vi "SPI Master and Slave with debug using PXI Trig [FPGA].vi"() -> ()   [LabVIEW 2019]
uses:
  <vilib>/Platform/TimedLoop/XDataNode/timing_clust.ctl
  <vilib>/Platform/TimedLoop/XDataNode/nitl_modes.ctl
  <vilib>/Platform/TimedLoop/XDataNode/wakeup.ctl
  SPI Master State.ctl
  SPI Slave State.ctl
  <vilib>/rvi/Emulation/niFpgaSctlEmulationGetInTimedLoop.vi
  <vilib>/rvi/Emulation/niFpgaEmulationReportErrorSimple.vi
  <vilib>/rvi/Emulation/niFpgaGetClockAttributes.vi
  <vilib>/rvi/Emulation/niFpgaCriticalErrorInLSC.vi
  <vilib>/rvi/eio/common/nirviEmuTemplateMethod_errors.vi
  <vilib>/rvi/interface/RandomDataEmulation/niFpgaRandomDataHandleErrors.vi
  <vilib>/Platform/TimedLoop/XDataNode/XDataNode.xnode
  <vilib>/eio/EIONode/EIONode.xnode
  <vilib>/rvi/DataTransferAndStorage/Container/XNode/niFpgaContainer.xnode
  <vilib>/rvi/interface/RandomDataEmulation/nirviRandomDataFpgaReadWriteTemplate.vi
  <vilib>/Platform/TimedLoop/XDataNode/XDNodeRunTimeDep.lvlib
panel:
  out "Slave Data Out":u32
  in  "Slave Data In":u32
  in  "Data Length":u8
  in  "HCP-1":u8
  out "Data Out":u32
  in  "Data In":u32
  in  "TX":bool
  in  "CPOL":bool
  in  "CPHA":bool
  in  "RESET":bool
  out "MISO":bool
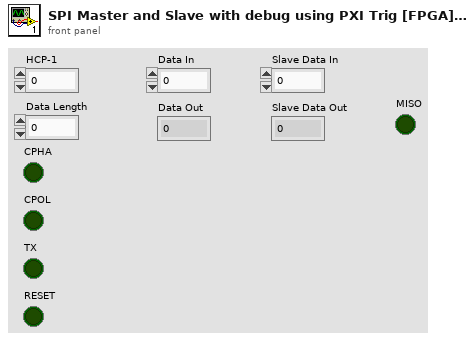
[diagram p1: front panel]
types:
  T1 = typedef "XDNodeRunTimeDep.lvlib/timing_clust.ctl" = cluster{"Expected End [f-1]":u64, "Actual End [f-1]":u64, "Finished Late? [f-1]":bool, "Expected End [i-1]":u64, "Actual End [i-1]":u64, "Finished Late? [i-1]":bool, "Expected Start [i]":u64, "Actual Start [i]":u64, "Expected Start [f]":u64, "Actual Start [f]":u64, "Source Name":string, "Structure Name":string, "Period":i64, "Deadline":i64, "Offset":i64, "Start":i64, "Priority":i32, "Timeout":i32, "Mode":T2, "Wakeup Reason":T3, "Error":errorcluster, "Source Type":string, "Secondary Source Type":string, "Global End Time":u64, "Global Start Time":u64, "Frame Duration":u64, "Iteration Duration":u64, "Assigned CPU":i32, "I/O Scan Engine Mode":u32}
  T2 = typedef "XDNodeRunTimeDep.lvlib/nitl_modes.ctl" = enum32{"No Change", "Process missed periods, maintain original phase", "Discard missed periods, maintain original phase", "Process missed periods, ignore original phase", "Discard missed periods, ignore original phase"}
  T3 = typedef "XDNodeRunTimeDep.lvlib/wakeup.ctl" = enum32{"Normal", "Aborted", "Asynchronous wakeup", "Timing source error", "Timed loop error", "Timeout"}
  T4 = typedef "SPI Slave State.ctl" = enum8{"RESET", "Wait for _SS", "Assert MISO", "Latch MOSI"}
  T5 = typedef "SPI Master State.ctl" = enum8{"RESET", "Wait for TX", "Assert MOSI", "Toggle SCLK", "Latch MISO and Toggle SCLK", "Assert MOSI and Toggle SCLK"}
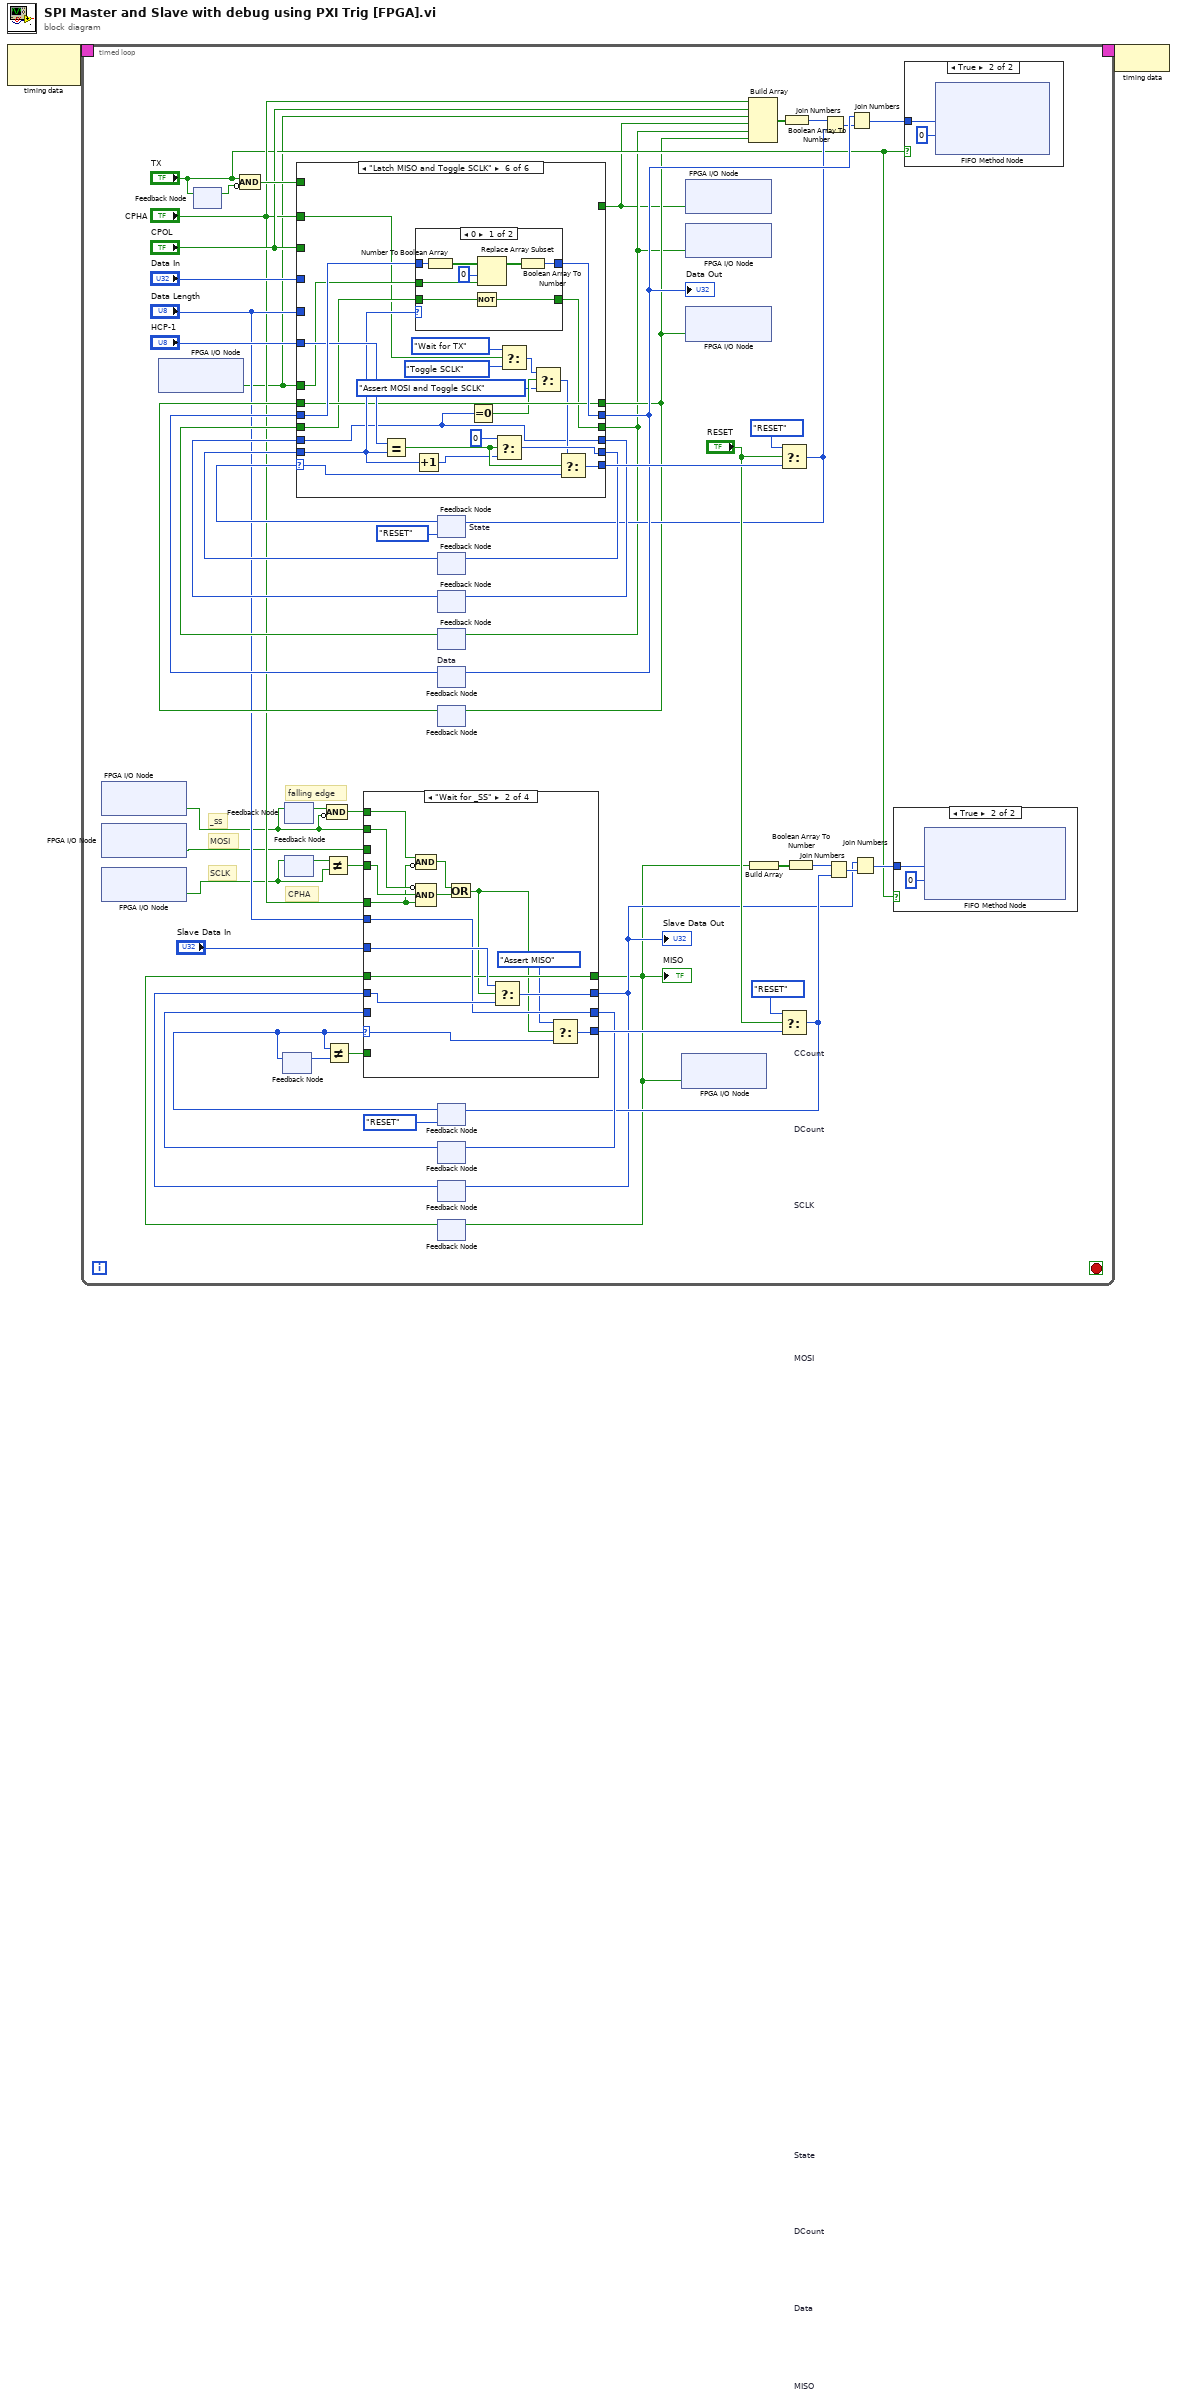
[diagram p0: block diagram]
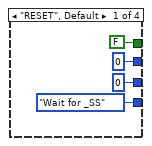
[diagram p3: hidden frame]
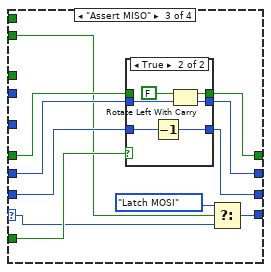
[diagram p4: hidden frame]
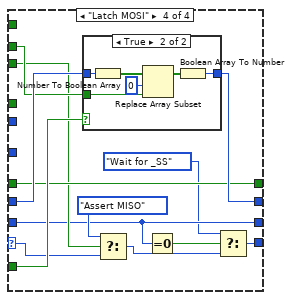
[diagram p6: hidden frame]
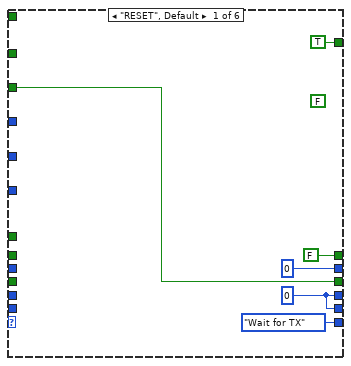
[diagram p9: hidden frame]
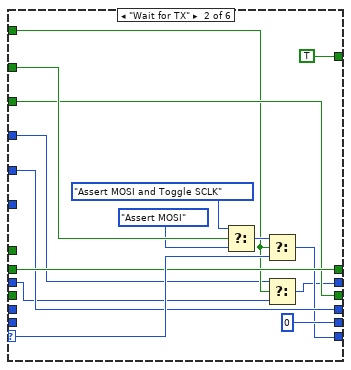
[diagram p10: hidden frame]
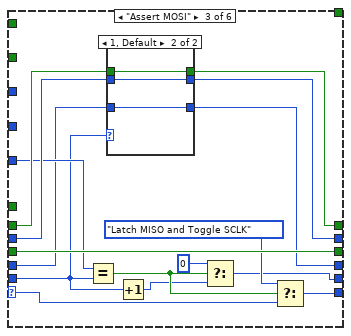
[diagram p11: hidden frame]
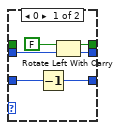
[diagram p12: hidden frame]
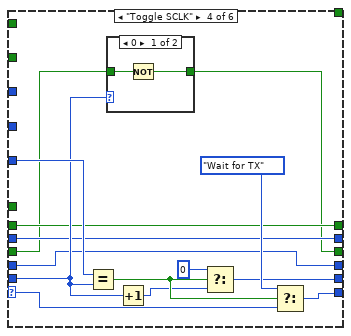
[diagram p13: hidden frame]
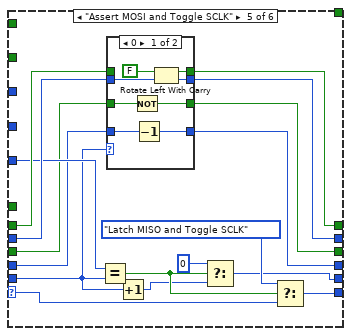
[diagram p15: hidden frame]
diagram:
  n1 = node-c288() -> (w2:T1)  [unwired: 1 in]
  n2 = timed-loop {
    timing: w2 -> [_]
    timing-out: [_] -> w1
    stop <- _ stop-if-true
    # "CPHA"
    # "falling edge"
    # "SCLK"
    # "MOSI"
    # "_SS"
    n3 = xnode "FPGA I/O Node"() -> ("PXI_Trig0"=w5:bool)  [unwired: 1 in, 1 out]
    n4 = xnode "FPGA I/O Node"() -> ("PXI_Trig2"=w4:bool)  [unwired: 1 in, 1 out]
    n5 = xnode "FPGA I/O Node"() -> ("PXI_Trig1"=w3:bool)  [unwired: 1 in, 1 out]
    n6 = xnode "FPGA I/O Node"() -> ("PXI_Trig3"=w9:bool)  [unwired: 1 in, 1 out]
    n7 = feedback #1() -> (w53:bool)  [unwired: 1 in]
    n8 = feedback-in #1("TX") -> ()
    n9 = Compound Arithmetic op=AND("TX", invert w53) -> (w45:bool)
    n10 = feedback #2 ("State")() -> (w20:T4)  [unwired: 1 in]
    n11 = feedback #3() -> (w24:bool)  [unwired: 1 in]
    n12 = feedback-in #3(w5) -> ()
    n13 = feedback #4() -> (w22:bool)  [unwired: 1 in]
    n14 = feedback-in #4(w3) -> ()
    n15 = Not Equal?(x=w22, y=w3) -> (x != y?=w21:bool)
    n16 = Compound Arithmetic op=AND(w24, invert w5) -> (w23:bool)
    n17 = feedback #5 "State"(SPI_Master_State."RESET") -> (w56:T5)
    n18 = feedback #6 "CCount"() -> (w50:u8)  [unwired: 1 in]
    n19 = feedback #7 "DCount"() -> (w49:u8)  [unwired: 1 in]
    n20 = feedback #8 "SCLK"() -> (w48:bool)  [unwired: 1 in]
    n21 = feedback #9 "Data"() -> (w46:u32)  [unwired: 1 in]
    n22 = feedback #10 "MOSI"() -> (w44:bool)  [unwired: 1 in]
    n23 = case shown="\"Latch MISO and Toggle SCLK\"" w56 {
      selector: w56 -> [_ w138 w150 w178 w194 w230]
      tunnel: [SPI_Master_State."Wait for TX" w131 w151 w179 w195 w231] -> w55
      tunnel: w45 -> [_ w130 _ _ _ _]
      tunnel: [w125 u8 0 w144 w172 w188 w225] -> w52
      tunnel: [w125 w133 w142 w171 w184 w213] -> w51
      tunnel: w50 -> [_ _ w147 w175 w191 w228]
      tunnel: w49 -> [_ _ w143 w171 w185 w213]
      tunnel: [TRUE ("MOSI") TRUE ("MOSI") _ _ _ _] -> w6
      tunnel: "CPHA" -> [_ w139 _ _ _ w219]
      tunnel: [w123 w132 w153 w167 w186 w221] -> w7
      tunnel: "CPOL" -> [w123 w132 _ _ _ _]
      tunnel: w48 -> [_ _ w153 w168 w187 w222]
      tunnel: "Data In" -> [_ w129 _ _ _ _]
      tunnel: [u32 0 ("Data In") w127 w156 w170 w199 w233] -> w38
      tunnel: w46 -> [_ w128 w157 w170 w200 w234]
      tunnel: "HCP-1" -> [_ _ w152 w180 w196 w232]
      tunnel: w9 -> [_ _ _ _ _ w223]
      tunnel: "Data Length" -> [_ w133 _ _ _ _]
      tunnel: [FALSE ("msb carry out") w134 w155 w169 w198 w224] -> w8
      tunnel: w44 -> [_ w134 w154 w169 w197 w224]
      frame "RESET", Default {
        (unwired) FALSE ("msb carry out")
        w125 = u8 0
      }
      frame "Wait for TX" {
        n24 = Select(t=SPI_Master_State."Assert MOSI and Toggle SCLK", s=w139, f=SPI_Master_State."Assert MOSI" ("t")) -> (s? t:f=w135:T5)
        n25 = Select(t=w135, s=w130, f=w138) -> (s? t:f=w131:T5)
        n26 = Select(t=w129, s=w130, f=w128) -> (s? t:f=w127:u32)
      }
      frame "Assert MOSI" {
        n27 = Equal?(x=w152, y=w147) -> (x = y?=w148:bool)
        n28 = case shown="1, Default" w147 {
          tunnel: w157 -> [w162 w165]
          tunnel: [w161 w165] -> w156
          tunnel: [w160 w166] -> w155
          tunnel: w154 -> [_ w166]
          tunnel: w143 -> [w159 w164]
          tunnel: [w158 w164] -> w142
          frame 0 {
            n29 = Decrement(x=w159) -> (x-1=w158:u8)
            n30 = Rotate Left With Carry(2:w162, 3:FALSE ("carry")) -> (0:w161:u32, 1:w160:bool)
          }
          frame 1, Default {
          }
        }
        n31 = Increment(x=w147) -> (x+1=w146:u8)
        n32 = Select(t=u8 0, s=w148, f=w146) -> (s? t:f=w144:u8)
        n33 = Select(t=SPI_Master_State."Latch MISO and Toggle SCLK", s=w148, f=w150) -> (s? t:f=w151:T5)
      }
      frame "Toggle SCLK" {
        n34 = Equal?(x=w180, y=w175) -> (x = y?=w176:bool)
        n35 = case shown="0" w175 {
          tunnel: w168 -> [w182 w183]
          tunnel: [w181 w183] -> w167
          frame 0 {
            n36 = Not(x=w182) -> (.not. x?=w181:bool)
          }
          frame 1, Default {
          }
        }
        n37 = Increment(x=w175) -> (x+1=w174:u8)
        n38 = Select(t=u8 0, s=w176, f=w174) -> (s? t:f=w172:u8)
        n39 = Select(t=SPI_Master_State."Wait for TX", s=w176, f=w178) -> (s? t:f=w179:T5)
      }
      frame "Assert MOSI and Toggle SCLK" {
        n40 = Equal?(x=w196, y=w191) -> (x = y?=w192:bool)
        n41 = case shown="0" w191 {
          tunnel: w200 -> [w207 w211]
          tunnel: [w206 w211] -> w199
          tunnel: [w205 w212] -> w198
          tunnel: w197 -> [_ w212]
          tunnel: w187 -> [w204 w210]
          tunnel: [w203 w210] -> w186
          tunnel: w185 -> [w202 w209]
          tunnel: [w201 w209] -> w184
          frame 0 {
            n42 = Not(x=w204) -> (.not. x?=w203:bool)
            n43 = Decrement(x=w202) -> (x-1=w201:u8)
            n44 = Rotate Left With Carry(2:w207, 3:FALSE ("carry")) -> (0:w206:u32, 1:w205:bool)
          }
          frame 1, Default {
          }
        }
        n45 = Increment(x=w191) -> (x+1=w190:u8)
        n46 = Select(t=u8 0, s=w192, f=w190) -> (s? t:f=w188:u8)
        n47 = Select(t=SPI_Master_State."Latch MISO and Toggle SCLK", s=w192, f=w194) -> (s? t:f=w195:T5)
      }
      frame "Latch MISO and Toggle SCLK" {
        n48 = Equal?(x=w232, y=w228) -> (x = y?=w229:bool)
        n49 = Increment(x=w228) -> (x+1=w227:u8)
        n50 = case shown="0" w228 {
          tunnel: w234 -> [w242 w244]
          tunnel: [w237 w244] -> w233
          tunnel: w223 -> [w240 _]
          tunnel: w222 -> [w236 w243]
          tunnel: [w235 w243] -> w221
          frame 0 {
            n51 = Number To Boolean Array(number=w242) -> (Boolean array=w241:bool[])
            n52 = Not(x=w236) -> (.not. x?=w235:bool)
            n53 = Replace Array Subset(array=w241, new element=w240, index=0) -> (w238:bool[])
            n54 = Boolean Array To Number(Boolean array=w238) -> (number=w237:u32)
          }
          frame 1, Default {
          }
        }
        n55 = Equal To 0?(x=w213) -> (x = 0?=w220:bool)
        n56 = Select(t=u8 0, s=w229, f=w227) -> (s? t:f=w225:u8)
        n57 = Select(t=SPI_Master_State."Wait for TX", s=w219, f=SPI_Master_State."Toggle SCLK" ("t")) -> (s? t:f=w215:T5)
        n58 = Select(t=w215, s=w220, f=SPI_Master_State."Assert MOSI and Toggle SCLK" ("t")) -> (s? t:f=w217:T5)
        n59 = Select(t=w217, s=w229, f=w230) -> (s? t:f=w231:T5)
      }
    }
    "Data Out" <- w38
    n60 = feedback-in #6(w52) -> ()
    n61 = feedback-in #7(w51) -> ()
    n62 = feedback-in #8(w7) -> ()
    n63 = feedback-in #9(w38) -> ()
    n64 = feedback-in #10(w8) -> ()
    n65 = feedback #11 "State"(SPI_Slave_State."RESET" ("SPI Slave State")) -> (w19:T4)
    n66 = feedback-in #2(w19) -> ()
    n67 = Not Equal?(x=w19, y=w20) -> (x != y?=w18:bool)
    n68 = feedback #12 "DCount"() -> (w32:u8)  [unwired: 1 in]
    n69 = feedback #13 "Data"() -> (w29:u32)  [unwired: 1 in]
    n70 = feedback #14 "MISO"() -> (w28:bool)  [unwired: 1 in]
    n71 = case shown="\"Wait for _SS\"" w19 {
      selector: w19 -> [_ w66 w82 w105]
      tunnel: w4 -> [_ _ _ w108]
      tunnel: [SPI_Slave_State."Wait for _SS" ("SPI Slave State") w71 w81 w102] -> w35
      tunnel: w5 -> [_ w78 _ _]
      tunnel: w32 -> [_ _ w86 w101]
      tunnel: [u8 0 w72 w85 w101] -> w31
      tunnel: [u32 0 ("Data In") w74 w84 w109] -> w11
      tunnel: w29 -> [_ w73 w88 w111]
      tunnel: w28 -> [_ w69 w87 w107]
      tunnel: [FALSE ("msb carry out") w69 w83 w107] -> w10
      tunnel: "Data Length" -> [_ w72 _ _]
      tunnel: "Slave Data In" -> [_ w75 _ _]
      tunnel: "CPHA" -> [_ w64 _ _]
      tunnel: w23 -> [_ w76 _ _]
      tunnel: w21 -> [_ w77 w80 w106]
      tunnel: w18 -> [_ _ w89 w110]
      frame "RESET", Default {
      }
      frame "Wait for _SS" {
        n72 = Compound Arithmetic op=AND(w76, invert w64) -> (w67:bool)
        n73 = Compound Arithmetic op=AND(invert w78, w77, w64) -> (w70:bool)
        n74 = Or(x=w67, y=w70) -> (x .or. y?=w65:bool)
        n75 = Select(t=w75, s=w65, f=w73) -> (s? t:f=w74:u32)
        n76 = Select(t=SPI_Slave_State."Assert MISO", s=w65, f=w66) -> (s? t:f=w71:T4)
      }
      frame "Assert MISO" {
        n77 = case shown="True" w89 {
          tunnel: w88 -> [w91 w97]
          tunnel: [w91 w96] -> w84
          tunnel: [w92 w95] -> w83
          tunnel: w87 -> [w92 _]
          tunnel: w86 -> [w90 w94]
          tunnel: [w90 w93] -> w85
          frame False {
          }
          frame True {
            n78 = Decrement(x=w94) -> (x-1=w93:u8)
            n79 = Rotate Left With Carry(2:w97, 3:FALSE ("carry")) -> (0:w96:u32, 1:w95:bool)
          }
        }
        n80 = Select(t=SPI_Slave_State."Latch MOSI", s=w80, f=w82) -> (s? t:f=w81:T4)
      }
      frame "Latch MOSI" {
        n81 = case shown="True" w110 {
          tunnel: w111 -> [w112 w118]
          tunnel: [w112 w113] -> w109
          tunnel: w108 -> [_ w116]
          frame False {
          }
          frame True {
            n82 = Number To Boolean Array(number=w118) -> (Boolean array=w117:bool[])
            n83 = Replace Array Subset(array=w117, new element=w116, index=0) -> (w114:bool[])
            n84 = Boolean Array To Number(Boolean array=w114) -> (number=w113:u32)
          }
        }
        n85 = Select(t=SPI_Slave_State."Assert MISO", s=w106, f=w105) -> (s? t:f=w103:T4)
        n86 = Equal To 0?(x=w101) -> (x = 0?=w100:bool)
        n87 = Select(t=SPI_Slave_State."Wait for _SS", s=w100, f=w103) -> (s? t:f=w102:T4)
      }
    }
    "MISO" <- w10
    "Slave Data Out" <- w11
    n88 = feedback-in #12(w31) -> ()
    n89 = feedback-in #13(w11) -> ()
    n90 = feedback-in #14(w10) -> ()
    n91 = xnode "FPGA I/O Node"("PXI_Trig3"=w10) -> ()  [unwired: 1 in, 1 out]
    n92 = xnode "FPGA I/O Node"("PXI_Trig0"=w6) -> ()  [unwired: 1 in, 1 out]
    n93 = xnode "FPGA I/O Node"("PXI_Trig1"=w7) -> ()  [unwired: 1 in, 1 out]
    n94 = xnode "FPGA I/O Node"("PXI_Trig2"=w8) -> ()  [unwired: 1 in, 1 out]
    n95 = Build Array("CPHA", "CPOL", w9, w6, w7, w8) -> (w40:bool[])
    n96 = Build Array(w10) -> (w15:bool[])
    n97 = Select(t=SPI_Master_State."RESET", s="RESET", f=w55) -> (s? t:f=w30:T5)
    n98 = feedback-in #5(w30) -> ()
    n99 = Select(t=SPI_Slave_State."RESET", s="RESET", f=w35) -> (s? t:f=w13:T4)
    n100 = feedback-in #11(w13) -> ()
    n101 = Boolean Array To Number(Boolean array=w40) -> (number=w39:u8)
    n102 = Boolean Array To Number(Boolean array=w15) -> (number=w16:u8)
    n103 = Join Numbers(hi=w39, lo=w30) -> ((hi.lo)=w37:u16)
    n104 = Join Numbers(hi=w16, lo=w13) -> ((hi.lo)=w17:u16)
    n105 = Join Numbers(hi=w38, lo=w37) -> ((hi.lo)=w42:u64)
    n106 = Join Numbers(hi=w11, lo=w17) -> ((hi.lo)=w14:u64)
    n107 = case shown="True" "TX" {
      tunnel: w14 -> [_ w58]
      frame False {
      }
      frame True {
        n108 = xnode ("FIFO Method Node")("Element"=w58, "Timeout"=0) -> ()  [unwired: 1 in, 2 out]
      }
    }
    n109 = case shown="True" "TX" {
      tunnel: w42 -> [_ w119]
      frame False {
      }
      frame True {
        n110 = xnode ("FIFO Method Node")("Element"=w119, "Timeout"=0) -> ()  [unwired: 1 in, 2 out]
      }
    }
  }
  n111 = node-c288(w1) -> ()
